vi "Main.vi"() -> ()   [LabVIEW 2019]
doc: "The myRIO Project template acquires acceleration data from the onboard accelerometer and displays the changes of acceleration values in a waveform chart."
uses:
  <vilib>/myRIO/Instrument Drivers/Onboard IO/UART/typedef/VISA Configuration.ctl
  <vilib>/Instr/_visa.llb/VISA Configure Serial Port (Instr).vi
  <vilib>/myRIO/Express VI/Onboard IO/UART/UART Express VI.xnode
  <vilib>/myRIO/Instrument Drivers/Onboard IO/UART/UART.lvlib
panel:
  out "Read":string
  out "error out":errorcluster
  out "Character count":dbl
  in  "String":string
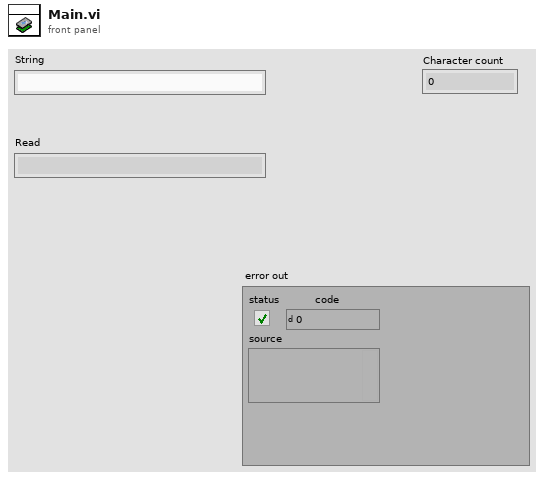
[diagram p1: front panel]
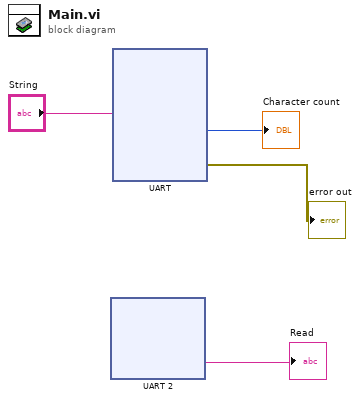
[diagram p0: block diagram]
diagram:
  n1 = xnode "UART 2"() -> ("Characters Read"=→"Read":string)  [unwired: 1 in, 1 out]
  n2 = xnode "UART"("Characters to Write"="String") -> ("Character Count"=→"Character count":u32, "error out"=→"error out":errorcluster)  [unwired: 1 in]
